vi "CMD_Lift.vi"(1 "Line":string) -> (0 "Done":bool)   [LabVIEW 2014]
uses:
  AppleScript Global Data.vi
panel:
  in  "Parameters":i32[](array[numeric])=[1, 1, 0, 1]
  in  "Subcommands":string[](array[string])=["at", "to", "tote", "until"]
  # "e"
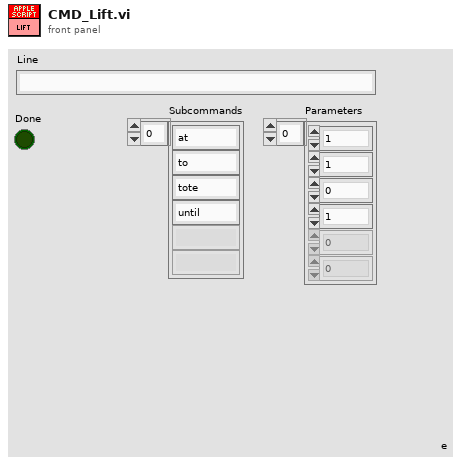
[diagram p1: front panel]
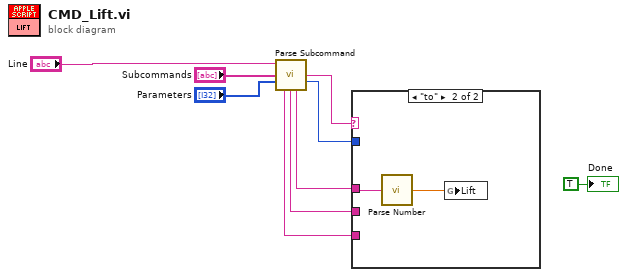
[diagram p0: block diagram]
diagram:
  n1 = call "Parse Subcommand.vi"("Text In"="Line", "Subcommands"="Subcommands", "Parameters"="Parameters") -> ("Subcommand"=w6:string, "# of Parameters"=w5:i32, "Parameter 3"=w2:string, "Parameter 2"=w3:string, "Parameter 1"=w4:string)  [unwired: 6 in, 2 out]
  n2 = case shown="\"to\"" w6 {
    tunnel: w5 -> [_ _]
    tunnel: w4 -> [_ w11]
    tunnel: w3 -> [_ _]
    tunnel: w2 -> [_ _]
    frame Default {
    }
    frame "to" {
      n3 = call "Parse Number.vi"("String"=w11) -> ("Number"=w10:dbl)
      n4 = global write "AppleScript Global Data.vi" "Lift"(w10) -> ()
    }
  }
  "Done" <- TRUE ("Done")
